vi "onStop.vi"(8 "error in (no error)":errorcluster, 11 "SMO":refnum<class "SMO.lvclass">) -> (0 "error out":errorcluster, 3 "SMO out":refnum<class "SMO.lvclass">)   [LabVIEW 2013, in "SMO.lvclass"]
uses:
  SMO.lvclass
  SMO.lvclass/SMO.ctl
  Typedefs/SMO Dependency--Cluster.ctl
  Support/Attribute.Owner/Attribute.Owner.lvclass
panel:
  # "For instructions on how to use the JKI State Machine Objects, examples and video tutorials, visit:\nhttp://jki.net/state-machine-objects/\n\nJKI State Machine Objects™\nhttp://jki.net/state-machine-objects/\nCopyright (C) 2005-2015, JKI <info@jki.net>\nALL RIGHTS RESERVED"
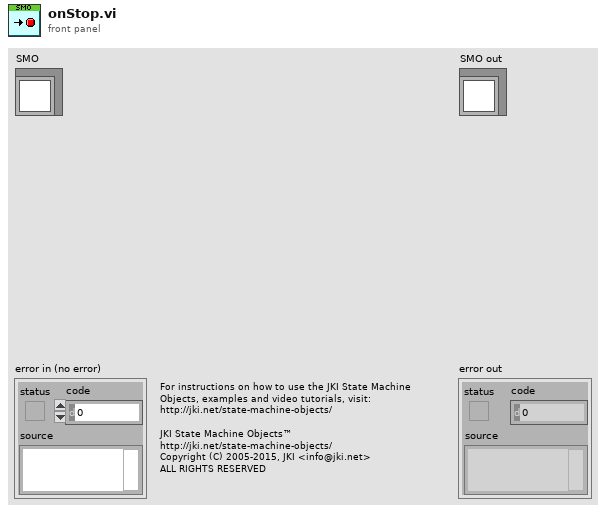
[diagram p1: front panel]
types:
  T1 = typedef "SMO.lvclass/SMO Dependency--Cluster.ctl" = cluster{"Dependency":refnum<class "SMO.lvclass">, "Level":string}
  T2 = typedef "SMO.lvclass/PrivateData--Ref.ctl" = refnum<data-value>
  T3 = typedef "SMO.lvclass/PrivateData--Cluster.ctl" = cluster{"Parent Call":T4, "Registered Processes":T5[], "Sync Notifier":refnum<notifier>, "Process Error Notifier":refnum<notifier>, "Protected Events":T6, "Public Events":T7, "SMO State":T8, "[Dependencies]":T1[], "[Attributes]":refnum<class "Attribute.lvclass">[], "Launcher Close":refnum<notifier>}
  T4 = typedef "SMO.lvclass/Parent Call--Enum.ctl" = enum16{"Allows parent to run", "Does not request parent to run"}
  T5 = typedef "SMO.lvclass/RegisteredProcessData--Cluster.ctl" = cluster{"Name":string, "Static VI Ref":refnum<vi>, "Running":bool, "NotifierRef":u32}
  T6 = typedef "SMO.lvclass/Protected Events.ctl" = cluster{"StopProcesses":refnum<user-event>, "AbortProcesses":refnum<user-event>, "Config Changed":refnum<user-event>}
  T7 = typedef "SMO.lvclass/Public Events.ctl" = cluster{"Error":refnum<user-event>, "State":refnum<user-event>}
  T8 = typedef "SMO.lvclass/SMOState --Enum.ctl" = enum16{"unknown", "Created", "Started", "Stopped"}
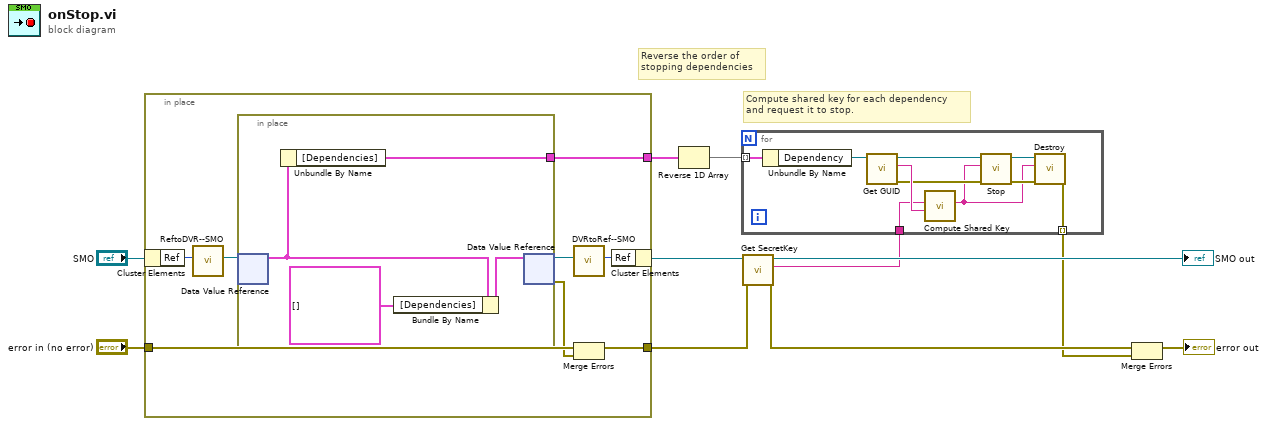
[diagram p0: block diagram]
diagram:
  # "Reverse the order of\nstopping dependencies"
  # "Compute shared key for each dependency\nand request it to stop."
  n1 = in-place {
    in-place-border: "error in (no error)" -> [w15]
    in-place-border: [w13] -> w4
    in-place-border: [w12] -> w8
    n2 = in-place-cluster #1("SMO") -> ("Ref"=w19:u32)
    n3 = call "ReftoDVR--SMO.vi"("Ref"=w19) -> ("Ref"=w18:T2)  [unwired: 10 in]
    n4 = in-place {
      in-place-border: [w23] -> w12
      n5 = in-place-dvr #2(w18) -> (w22:T3)  [unwired: 1 out]
      n6 = Unbundle By Name(w22) -> ("[Dependencies]"=w23:T1[])
      n7 = Bundle By Name(cluster=w22, "[Dependencies]"=T1[] []) -> (w21:T3)
      n8 = in-place-dvr #2(w21) -> (w17:T2, w14:errorcluster)
    }
    n9 = call "DVRtoRef--SMO.vi"("Ref"=w17) -> ("Ref"=w16:u32)  [unwired: 10 in]
    n10 = Merge Errors(w15, w14) -> (w13:errorcluster)
    n11 = in-place-cluster #1("Ref"=w16) -> (w7:refnum<class "SMO.lvclass">)
  }
  n12 = Reverse 1D Array(array=w8) -> (reversed array=w2:T1[])
  n13 = call "Get SecretKey.vi"("error in (no error)"=w4, "SMO"=w7) -> ("error out"=w5:errorcluster, "SecretKey"=w3:string, "SMO out"=→"SMO out":refnum<class "SMO.lvclass">)  [unwired: 7 in]
  n14 = for {
    tunnel: w2 -> [w27] mode=indexing
    tunnel: w3 -> [w29]
    tunnel: [w24] -> w1 mode=indexing
    n15 = Unbundle By Name(w27) -> ("Dependency"=w26:refnum<class "SMO.lvclass">)
    n16 = call "Get GUID.vi"("SMO"=w26) -> ("error out"=w28:errorcluster, "GUID"=w30:string, "SMO out"=w31:refnum<class "SMO.lvclass">)  [unwired: 8 in]
    n17 = call "Compute Shared Key.vi"("GUID"=w30, "SecretKey"=w29) -> ("Shared Key"=w25:string)  [unwired: 9 in]
    n18 = call "Stop.vi"("error in (no error)"=w28, "Shared Key"=w25, "SMO"=w31) -> ("error out"=w33:errorcluster, "SMO out"=w32:refnum<class "SMO.lvclass">)  [unwired: 7 in]
    n19 = call "Destroy.vi"("error in (no error)"=w33, "Shared Key"=w25, "SMO"=w32) -> ("error out"=w24:errorcluster)  [unwired: 8 in]
  }
  n20 = Merge Errors(w5, w1) -> (→"error out":errorcluster)
